vi "Drive Power.vi"(4 "invertPower":bool[](array[boolean])) -> (5 "drivePower":dbl[](array[numeric]))   [LabVIEW 2019]
uses:
  swerveData.vi
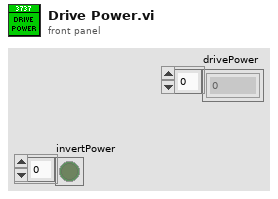
[diagram p1: front panel]
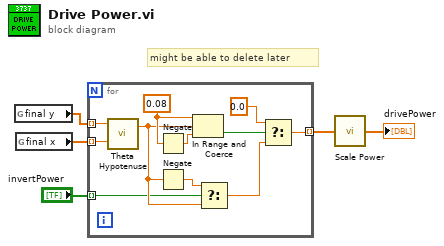
[diagram p0: block diagram]
diagram:
  # "might be able to delete later"
  n1 = global read "swerveData.vi" "final y"() -> (w5:dbl[])
  n2 = global read "swerveData.vi" "final x"() -> (w4:dbl[])
  n3 = for {
    tunnel: w5 -> [w16] mode=indexing
    tunnel: w4 -> [w15] mode=indexing
    tunnel: "invertPower" -> [w7] mode=indexing
    tunnel: [w6] -> w3 mode=indexing
    w13 = 0.08 ("upper limit")
    n4 = call "Theta Hypotenuse.vi"("x value"=w15, "y value"=w16) -> ("Hypotenuse"=w9:dbl)  [unwired: 1 out]
    n5 = Negate(x=w13) -> (-x=w14:dbl)
    n6 = Negate(x=w9) -> (-x=w10:dbl)
    n7 = In Range and Coerce(upper limit=w13, x=w9, lower limit=w14) -> (In Range?=w12:bool)  [unwired: 1 out]
    n8 = Select(t=w10, s=w7, f=w9) -> (s? t:f=w8:dbl)
    n9 = Select(t=0.0, s=w12, f=w8) -> (s? t:f=w6:dbl)
  }
  n10 = call "Scale Power.vi"("inputPower"=w3) -> ("outputPower"=→"drivePower":dbl[])
